vi "AuMT8852B Tester Bluetooth Address.vi"(8 "error in (no error)":errorcluster, 11 "VISA session":refnum<visa-resource-name>) -> (0 "error out":errorcluster, 2 "error code":i32, 3 "VISA session out":refnum<visa-resource-name>, 4 "Tester Bluetooth address out":string)   [LabVIEW 2017]
doc: "Anritsu MT8852B Bluetooth Tester\n\nRetrieves the Bluetooth address of the MT8850.\n\nOUTPUTS\nTester bluetooth address out - the current tester bluetooth address."
uses:
  <instrlib>/aumt8852B/General/Utilities/MT8850 Attribute ID.ctl
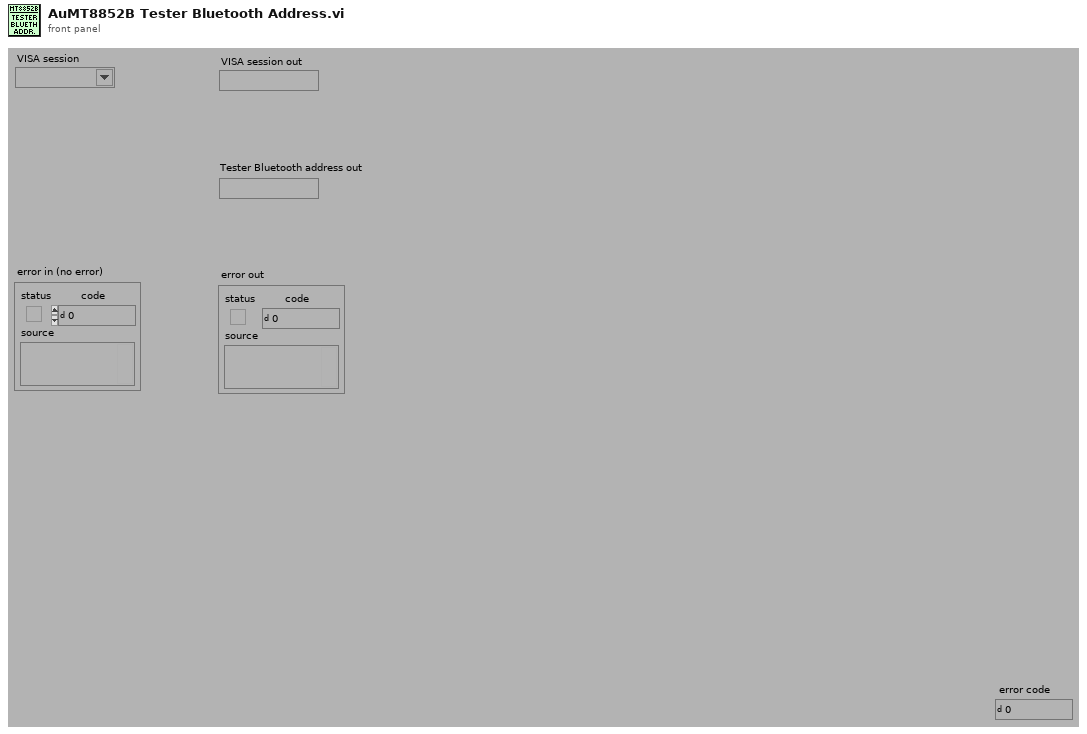
[diagram p1: front panel]
types:
  T1 = typedef "MT8850 Attribute ID.ctl" = enum16{"Operation mode", "Selected script", "EUT address source", "EUT Address", "EUT HCI RS232 Baud Rate", "Tester GPIB Address", "Tester RS232 Baud Rate", "Tester Bluetooth Address", "Tester Contrast", "Tester Key Click On", "Tester Modulation Index", "Tester Poll-Null Mode", "Tester Power Range", "Tester RS232 Mode", "Beep on Illegal Entry", "Display User Text", "User Text", "Calibration TX Modulation DAC", "Calibration RX Channel", "Calibration TX Channel", "Calibration TX Power", "Calibration Use TX Table", "Inquiry Request User-friendly Name", "Inquiry Number of Responses", "Inquiry Timeout", "Script Frequency Display", "Script Loop Count", "Script Loop Continuously", "Script Loop Stop on Fail", "Link timeout", "Page timeout", "Filter bandwidth", "SCO air code", "SCO bit position", "SCO input code", "SCO input data", "SCO input sample size", "SCO loopback mode", "SCO packet type", "SCO tone generator", "Tester page scan repetition mode", "Tester follow test mode", "Tester authentication state", "Tester authentication pin code", "Tester authentication pin length"}
  T2 = typedef "Attribute Status.ctl" = enum16{"No I/O needed", "I/O needed"}
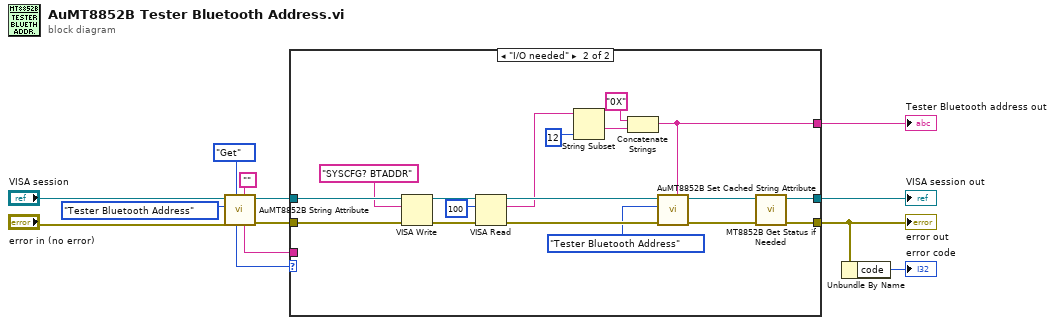
[diagram p0: block diagram]
diagram:
  n1 = call <instrlib>:"AuMT8852B String Attribute.vi"("Value (\"\")"="", "Set/Get (Set)"=enum16{"Set", "Get"}."Get", "error in (no error)"="error in (no error)", "Attribute ID"=MT8850_Attribute_ID."Tester Bluetooth Address", "VISA session"="VISA session") -> ("error out"=w9:errorcluster, "VISA session out"=w10:refnum<visa-resource-name>, "Value out"=w12:string, "Status"=w8:T2)  [unwired: 3 in]
  n2 = case shown="\"I/O needed\"" w8 {
    tunnel: w12 -> [w16 _]
    tunnel: [w14 w28] -> w1
    tunnel: [w15 w29] -> w11
    tunnel: w10 -> [w15 w34]
    tunnel: w9 -> [w14 w33]
    tunnel: [w16 w32] -> w7
    frame "No I/O needed", Default {
    }
    frame "I/O needed" {
      n3 = VISA Write(VISA resource name=w34, write buffer="SYSCFG? BTADDR" ("write buffer (\"\")"), error in (no error)=w33) -> (VISA resource name out=w27:refnum<visa-resource-name>, error out=w24:errorcluster)  [unwired: 1 out]
      n4 = VISA Read(VISA resource name=w27, byte count=u32 100 ("byte count (0)"), error in (no error)=w24) -> (VISA resource name out=w23:refnum<visa-resource-name>, read buffer=w20:string, error out=w22:errorcluster)  [unwired: 1 out]
      n5 = String Subset(string=w20, length (rest)=12) -> (substring=w18:string)  [unwired: 1 in]
      n6 = Concatenate Strings("0X", w18) -> (w32:string)
      n7 = call <instrlib>:"AuMT8852B Set Cached String Attribute.vi"("Value (\"\")"=w32, "error in (no error)"=w22, "Attribute ID"=MT8850_Attribute_ID."Tester Bluetooth Address", "VISA session"=w23) -> ("error out"=w30:errorcluster, "VISA session out"=w31:refnum<visa-resource-name>)  [unwired: 6 in]
      n8 = call <instrlib>:"MT8852B Get Status if Needed.vi"("error in (no error)"=w30, "VISA session"=w31) -> ("error out"=w28:errorcluster, "VISA session out"=w29:refnum<visa-resource-name>)  [unwired: 8 in]
    }
  }
  "error out" <- w1
  "VISA session out" <- w11
  "Tester Bluetooth address out" <- w7
  n9 = Unbundle By Name(w1) -> ("code"=→"error code":i32)
